vi "Think.vi"(0 "X":i8, 1 "Y":i8, 2 "Sensor View":i8[][](array[numeric]), 3 "Sense Heading":i8, 4 "E":i8) -> (5 "V Heading":i8)   [LabVIEW 2014]
doc: "This VI takes in the current location of the robot (X,Y), the 3x3 sensor reading of the surrounding area, and the direction of the highest-valued neighboring food source."
panel:
  # "Vcode\n  6 7 8\n  5 0 1\n  4 3 2"
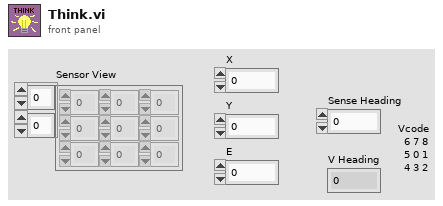
[diagram p1: front panel]
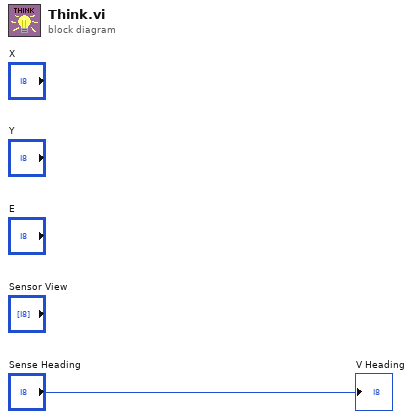
[diagram p0: block diagram]
diagram:
  "V Heading" <- "Sense Heading"
